vi "rotate face.vi"(10 "Face to act on":i32, 11 "Direction":T1=enum."Right") -> (2 "To":cluster{"row":i32, "column":i32}[](array[cluster]), 3 "From":cluster{"row":i32, "column":i32}[](array[cluster]))   [LabVIEW 2019]
uses:
  section movement.ctl
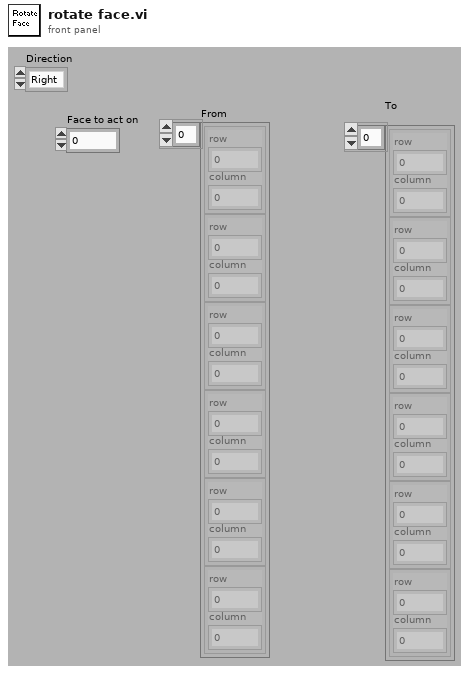
[diagram p1: front panel]
types:
  T1 = typedef "section movement.ctl" = enum16{"Left", "Right"}
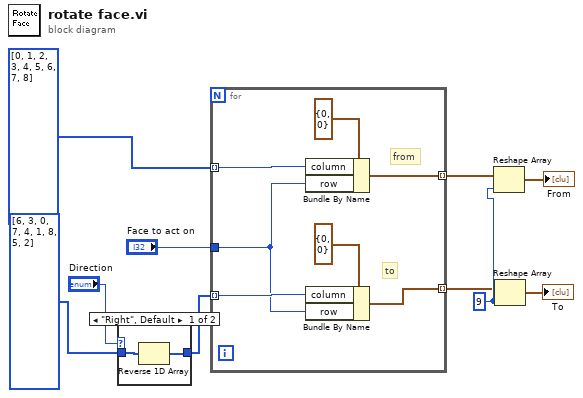
[diagram p0: block diagram]
diagram:
  w9 = 9 ("dimension size")
  n1 = case shown="\"Right\", Default" "Direction" {
    tunnel: i32[] [6, 3, 0, 7, 4, 1, 8, 5, 2] -> [w12 w13]
    tunnel: [w11 w13] -> w2
    frame "Right", Default {
      n2 = Reverse 1D Array(array=w12) -> (reversed array=w11:i32[])
    }
    frame "Left" {
    }
  }
  n3 = for {
    tunnel: [w18] -> w5 mode=indexing
    tunnel: [w17] -> w6 mode=indexing
    tunnel: i32[] [0, 1, 2, 3, 4, 5, 6, 7, 8] -> [w16] mode=indexing
    tunnel: w2 -> [w15] mode=indexing
    tunnel: "Face to act on" -> [w14]
    # "from"
    # "to"
    n4 = Bundle By Name(cluster=cluster{"row":i32, "column":i32} {"row"=0, "column"=0} ("From"), "column"=w16, "row"=w14) -> (w18:cluster{"row":i32, "column":i32})
    n5 = Bundle By Name(cluster=cluster{"row":i32, "column":i32} {"row"=0, "column"=0} ("From"), "column"=w15, "row"=w14) -> (w17:cluster{"row":i32, "column":i32})
  }
  n6 = Reshape Array(w5, w9) -> (→"From":cluster{"row":i32, "column":i32}[])
  n7 = Reshape Array(w6, w9) -> (→"To":cluster{"row":i32, "column":i32}[])
